vi "testMain.vi"() -> ()   [LabVIEW 2016]
uses:
  <vilib>/FPGAPlugInAG/roboRIO/niLvFpga_Open_roboRIO.vi
  <vilib>/rvi/interface/common/dynamic/niFpgaDynamicAddResources.vi
  <vilib>/Utility/error.llb/Error Cluster From Error Code.vi
  <vilib>/rvi/errors/niLvFpgaAdjustHostInterfaceError.vi
  <vilib>/rvi/interface/nirviOpenFPGA/nirviOpenFPGA.xnode
  FPGA Bitfiles/nRF24Communicati_FPGATarget_FPGATest_lnf7SjQfCOM.lvbitx
  FPGATest.vi
  <vilib>/rvi/interface/nirviReadWriteControl/nirviReadWriteControl.xnode
  NiFpgaLv.dll
  <vilib>/rvi/interface/Simulation/niFpgaSimulationCallBeginRW.vi
panel:
  out "ByteOut":u8
  in  "ByteIn":u8
  in  "NewData":bool
  in  "stop":bool
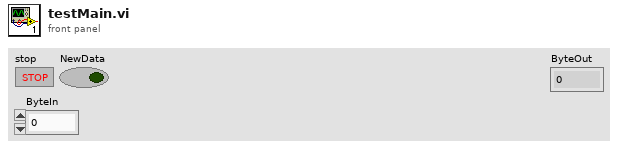
[diagram p1: front panel]
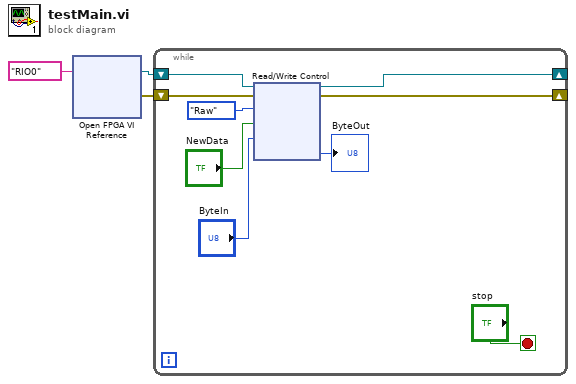
[diagram p0: block diagram]
diagram:
  n1 = xnode "Open FPGA VI Reference"("resource name"=tag "RIO0") -> ("FPGA VI Reference Out"=w1:refnum<k20>, "error out"=w2:errorcluster)  [unwired: 1 in]
  n2 = while {
    shift-right: [w10] -> _
    shift-left: w2 -> [w11]
    shift-right: [w8] -> _
    shift-left: w1 -> [w9]
    stop <- "stop" stop-if-true
    n3 = xnode "Read/Write Control"("FPGA VI Reference In"=w9, "error in"=w11, "Enum"=enum16{"ReadWrite", "Raw"}."Raw", "NewData"="NewData", "ByteIn"="ByteIn") -> ("FPGA VI Reference Out"=w8:refnum<k20>, "error out"=w10:errorcluster, "ByteOut"=→"ByteOut":u8)
  }
